vi "Subvi counter photons U8.vi"(6 "Pixel clock count":u16, 8 "Clock":bool, 9 "Single photon":bool) -> (1 "Photon count":u8)   [LabVIEW 2017]
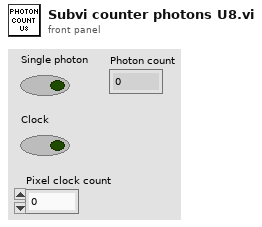
[diagram p1: front panel]
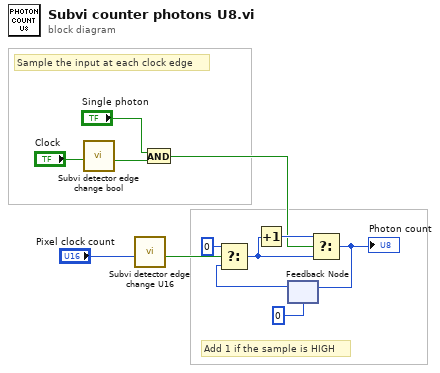
[diagram p0: block diagram]
diagram:
  # "Add 1 if the sample is HIGH"
  # "Sample the input at each clock edge"
  n1 = call "Subvi detector edge change bool.vi"("Input"="Clock") -> ("Output"=w6:bool)  [unwired: 8 in]
  n2 = call "Subvi detector edge change U16.vi"("Input"="Pixel clock count") -> ("Output"=w2:bool)  [unwired: 10 in]
  n3 = And(x="Single photon", y=w6) -> (x .and. y?=w3:bool)
  n4 = feedback #1(u8 0) -> (w8:u8)
  n5 = Select(t=u8 0, s=w2, f=w8) -> (s? t:f=w7:u8)
  n6 = Increment(x=w7) -> (x+1=w12:u8)
  n7 = Select(t=w12, s=w3, f=w7) -> (s? t:f=w9:u8)
  "Photon count" <- w9
  n8 = feedback-in #1(w9) -> ()
